vi "cargarDatoVarilla.vi"(11 "IndiceAUltimoValor\nAgregadoEnLaTabla":i32=1) -> ()   [LabVIEW 2014]
uses:
  claseVarilla/claseVarilla.lvclass
panel:
  out "dataReading":T1
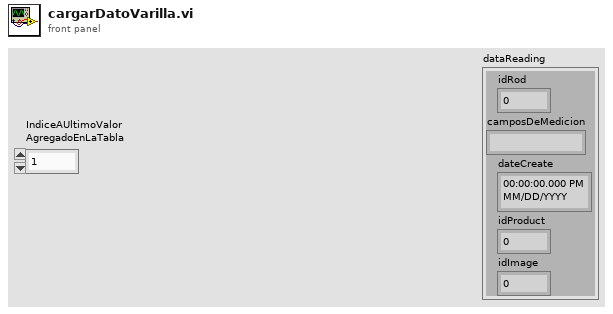
[diagram p1: front panel]
types:
  T1 = cluster{"idRod":dbl, "camposDeMedicion":string, "dateCreate":timestamp, "idProduct":dbl, "idImage":dbl}
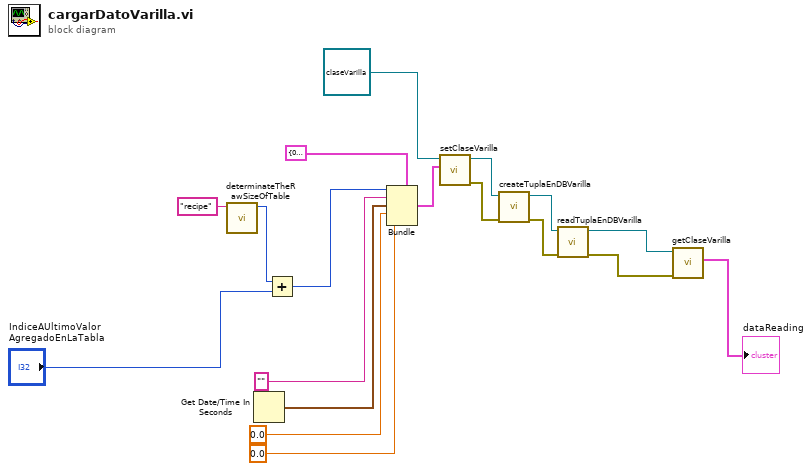
[diagram p0: block diagram]
diagram:
  n1 = call "determinateTheRawSizeOfTable.vi"("tableName"="recipe") -> ("sizeOfTableInNumberRaw"=w2:i32)  [unwired: 8 in, 1 out]
  n2 = Get Date/Time In Seconds() -> (seconds since 1Jan1904=w11:timestamp)
  n3 = Add(x=w2, y="IndiceAUltimoValor\nAgregadoEnLaTabla") -> (x+y=w13:i32)
  n4 = Bundle(cluster=T1 {"idRod"=0.0, "camposDeMedicion"="", "dateCreate"=timestamp(0 s since 1904-01-01), "idProduct"=0.0, "idImage"=0.0} ("dataToSet"), "idRod"=w13, "camposDeMedicion"="", "dateCreate"=w11, "idProduct"=0.0, "idImage"=0.0) -> (w15:T1)
  n5 = call "setClaseVarilla.vi"("dataToSet"=w15, "claseVarilla in"=refnum<class "claseVarilla.lvclass"> refnum ("claseVarilla.lvclass")) -> ("error out"=w7:errorcluster, "claseVarilla out"=w8:refnum<class "claseVarilla.lvclass">)  [unwired: 8 in]
  n6 = call "createTuplaEnDBVarilla.vi"("error in"=w7, "claseVarilla in"=w8) -> ("error out"=w5:errorcluster, "claseVarilla out"=w6:refnum<class "claseVarilla.lvclass">)  [unwired: 8 in]
  n7 = call "readTuplaEnDBVarilla.vi"("error in"=w5, "claseVarilla in"=w6) -> ("error out"=w3:errorcluster, "claseVarilla out"=w4:refnum<class "claseVarilla.lvclass">)  [unwired: 8 in]
  n8 = call "getClaseVarilla.vi"("error in"=w3, "claseVarilla in"=w4) -> ("dataReading"=→"dataReading":T1)  [unwired: 7 in, 2 out]
